vi "Sandbox.vi"() -> ()   [LabVIEW 2019, in "FPGA API Concrete.lvclass"]
uses:
  FPGA API Concrete.lvclass
  FPGA/TypeDef/DO index.ctl
  FPGA API Concrete.lvclass/FPGA API Concrete.ctl
  <vilib>/Utility/error.llb/Error Cluster From Error Code.vi
  <vilib>/rvi/errors/niLvFpgaAdjustHostInterfaceError.vi
  <vilib>/rvi/interface/nirviReadWriteControl/nirviReadWriteControl.xnode
  FPGA Ref.ctl
  <vilib>/ptbypt/NI_PtbyPt.lvlib
  NiFpgaLv.dll
  <vilib>/rvi/interface/Simulation/niFpgaSimulationCallBeginRW.vi
panel:
  in  "Mod5/AO1":fxp<+/-,20,5>
  out "Mod5/AO1 out":fxp<+/-,20,5>
  out "Ds":bool[](array[boolean])
  in  "#DO":T1 items=["DO 0 [KP1] [M12]", "DO 1 [ON KP2] [M21]", "DO 2 [ON KP3] [M24]", "DO 3 [WATER Y18.1 [DO3]]", "DO 4 [WATER Y18.2 [DO4]]", "DO 5 [KP6 Y29.1 33.7]", "DO 6 [KP7 Y29.2 33.8]", "DO 7 [KP8 Y29.3 33.9]", "DO 8 [KP9 Y29.4  33.12]", "DO 9 [KP10 Y29.5 33.1]", "DO 10 [KP11 Y29.6 33.2]", "DO 11 [KP12 Y29.7  33.13]", "DO 12 [KP13 Y29.8  33.11]", "DO 13 [KP14 Y29.9 33.10]", "DO 14 [KP15 Y29.10  33.6]", "DO 15 [KP16 Y29.11  33.5]", "DO 16 [KP17 Y29.12  33.4]", "DO 17 [KP18 Y29.13 33.3]", "DO 18 [AIR KP19]", "DO 19 [STEP DRIVE EN KP20]", "DO 20 [KP21 Y44.1 OPEN]", "DO 21 [ KP22 Y44.1 CLOSE]", "DO 22 [ KP23 Y44.2 OPEN]", "DO 23", "DO 24 [STEP DRIVE 1]", "DO 25 [STEP DRIVE 2]"]
  out "Numeric":i32
  out "avr %":dbl
  out "Raw %":dbl
  out "Waveform Chart":dbl[][](graph)
  out "DIs":bool[](array[boolean])
  out "dt(tiks) DI loop":u32
  out "dt(tiks) DO loop":u32
  out "dt(tiks) AI loop":u32
  out "error out":errorcluster
  in  "set":bool
  in  "Time uSec":u32
  in  "value":bool
  in  "stop":bool
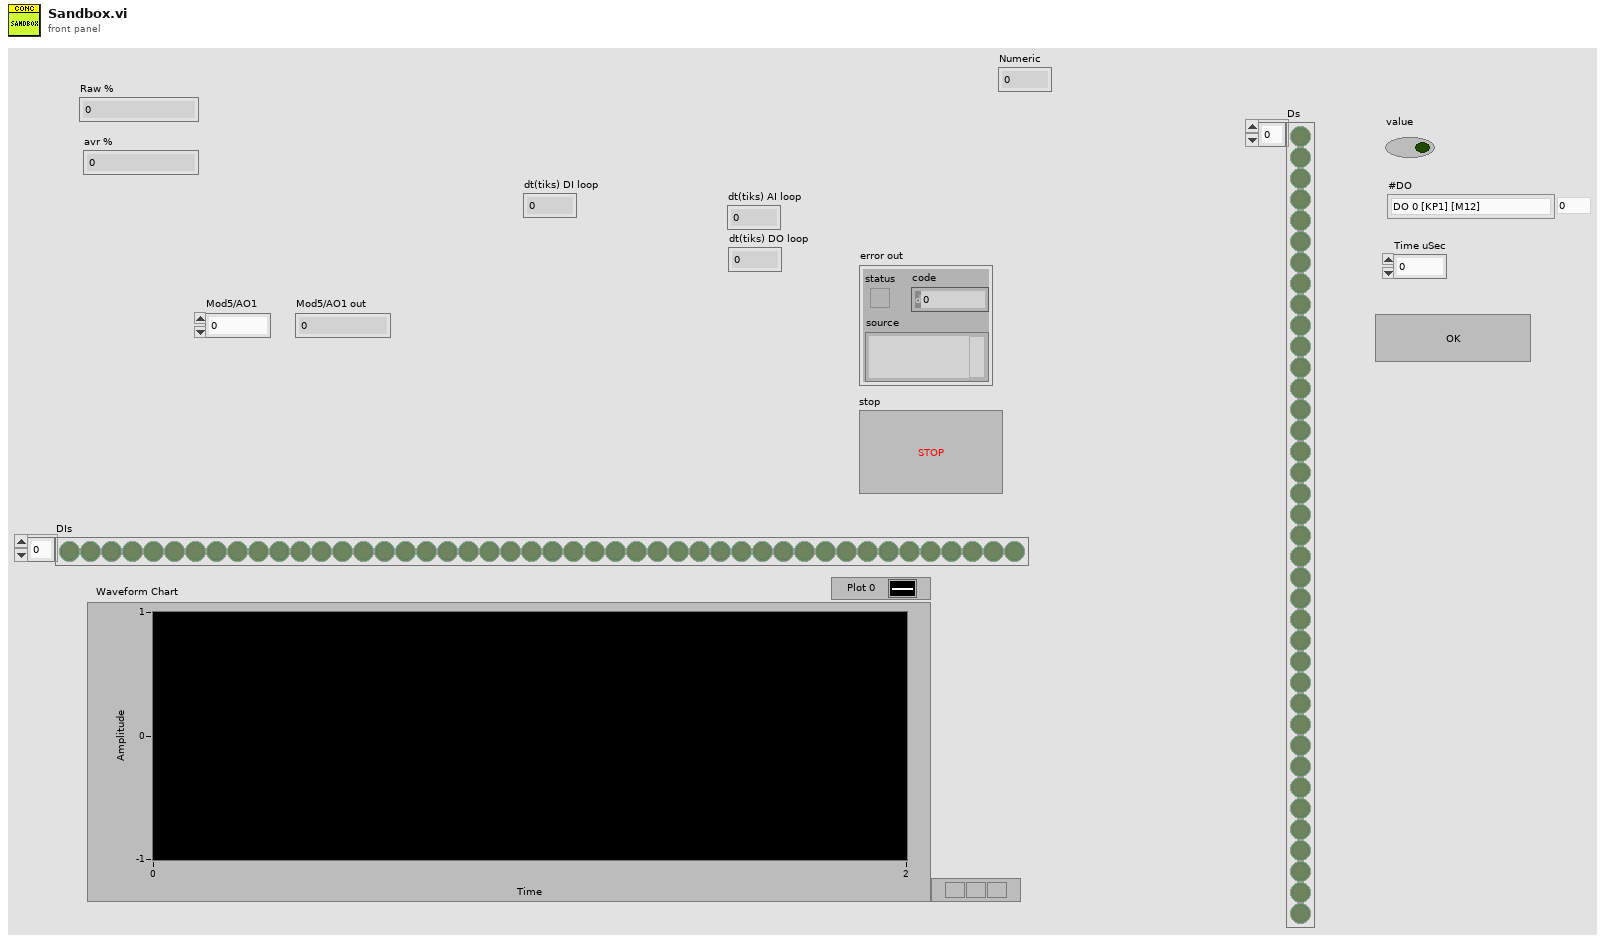
[diagram p1: front panel]
types:
  T1 = typedef "DO index.ctl" = u8
  T2 = typedef "FPGA API Concrete.lvclass/FPGA Ref.ctl" = refnum<k20>
  T3 = cluster{"AI_0 L5.1":fxp<+/-,21,-4>, "AI_1 T4.1":fxp<+/-,21,-4>, "AI_2 L5.2":fxp<+/-,21,-4>, "AI_3 T4.2":fxp<+/-,21,-4>, "AI_4 V":fxp<+/-,21,-4>, "AI_5 P38.1":fxp<+/-,21,-4>, "AI_6 P38.2":fxp<+/-,21,-4>, "AI_7 P38.3":fxp<+/-,21,-4>, "AI_8 P41.1":fxp<+/-,21,-4>, "AI_9 P41.2":fxp<+/-,21,-4>, "AI_10 P41.3":fxp<+/-,21,-4>, "AI_11":fxp<+/-,21,-4>, "AI_12":fxp<+/-,21,-4>, "AI_13":fxp<+/-,21,-4>, "AI_14":fxp<+/-,21,-4>, "AI_15":fxp<+/-,21,-4>}
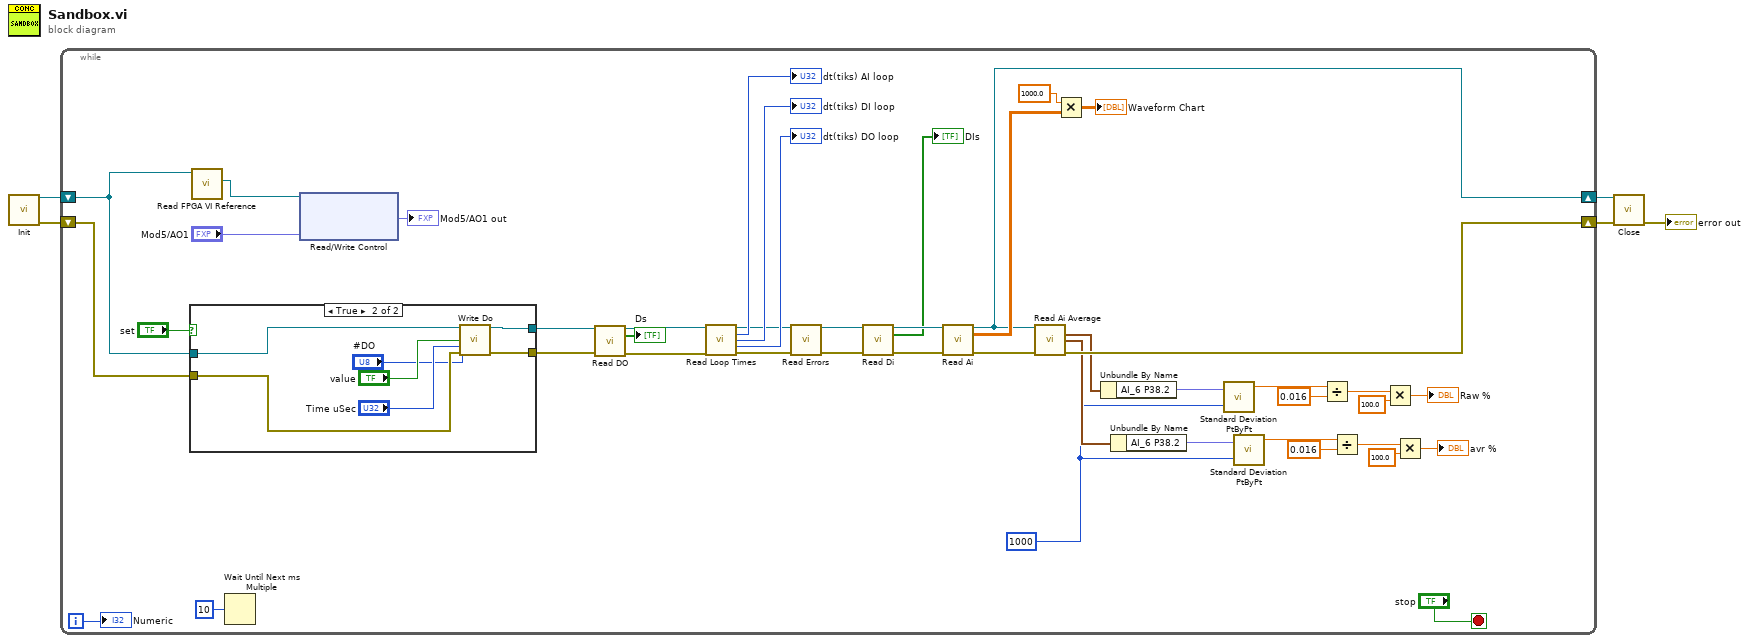
[diagram p0: block diagram]
diagram:
  n1 = call "Init.vi"() -> ("FPGA API out"=w5:refnum<class "FPGA API Concrete.lvclass">, "error out"=w4:errorcluster)  [unwired: 14 in]
  n2 = while {
    shift-right: [w34] -> w3
    shift-left: w5 -> [w9]
    shift-right: [w32] -> w2
    shift-left: w4 -> [w37]
    i -> [w16]
    stop <- "stop" stop-if-true
    w17 = 1000 ("sample length")
    n3 = case shown="True" "set" {
      tunnel: [w52 w59] -> w14
      tunnel: [w51 w58] -> w12
      tunnel: w9 -> [w52 w54]
      tunnel: w37 -> [w51 w57]
      frame False {
      }
      frame True {
        n4 = call-dynamic "Write Do.vi"("FPGA API in"=w54, "#DO"="#DO", "value"="value", "Time uSec"="Time uSec", "error in (no error)"=w57) -> ("FPGA API out"=w59:refnum<class "FPGA API Concrete.lvclass">, "error out"=w58:errorcluster)  [unwired: 9 in]
      }
    }
    n5 = call "Read FPGA VI Reference.vi"("FPGA API Concrete in"=w9) -> ("FPGA VI Reference"=w8:T2)  [unwired: 9 in, 1 out]
    n6 = Wait Until Next ms Multiple(millisecond multiple=u32 10) -> ()  [unwired: 1 out]
    n7 = xnode "Read/Write Control"("FPGA VI Reference In"=w8, "Mod5/AO1"="Mod5/AO1") -> ("Mod5/AO1 out"=→"Mod5/AO1 out":fxp<+/-,20,5>)  [unwired: 1 in, 2 out]
    n8 = call-dynamic "Read DO.vi"("FPGA API in"=w14, "error in (no error)"=w12) -> ("FPGA API out"=w13:refnum<class "FPGA API Concrete.lvclass">, "Ds"=→"Ds":bool[], "error out"=w11:errorcluster)  [unwired: 11 in]
    n9 = call-dynamic "Read Loop Times.vi"("FPGA API in"=w13, "error in (no error)"=w11) -> ("FPGA API out"=w43:refnum<class "FPGA API Concrete.lvclass">, "dt(tiks) AI loop"=→"dt(tiks) AI loop":u32, "dt(tiks) DI loop"=→"dt(tiks) DI loop":u32, "dt(tiks) DO loop"=→"dt(tiks) DO loop":u32, "error out"=w44:errorcluster)  [unwired: 8 in, 1 out]
    n10 = call-dynamic "Read Errors.vi"("FPGA API in"=w43, "error in (no error)"=w44) -> ("FPGA API out"=w42:refnum<class "FPGA API Concrete.lvclass">, "error out"=w41:errorcluster)  [unwired: 11 in, 1 out]
    n11 = call-dynamic "Read Di.vi"("FPGA API in"=w42, "error in (no error)"=w41) -> ("FPGA API out"=w39:refnum<class "FPGA API Concrete.lvclass">, "DIs"=→"DIs":bool[], "error out"=w40:errorcluster)  [unwired: 11 in]
    n12 = call-dynamic "Read Ai.vi"("FPGA API in"=w39, "error in (no error)"=w40) -> ("FPGA API out"=w34:refnum<class "FPGA API Concrete.lvclass">, "AI Data"=w36:dbl[][], "error out"=w33:errorcluster)  [unwired: 10 in, 1 out]
    n13 = call "Read Ai Average.vi"("FPGA API in"=w34, "error in (no error)"=w33) -> ("Raw"=w31:T3, "Average 1ms"=w18:T3, "error out"=w32:errorcluster)  [unwired: 10 in, 1 out]
    n14 = Multiply(x=1000.0, y=w36) -> (x*y=→"Waveform Chart":dbl[][])
    n15 = Unbundle By Name(w31) -> ("AI_6 P38.2"=w30:fxp<+/-,21,-4>)
    n16 = Unbundle By Name(w18) -> ("AI_6 P38.2"=w19:fxp<+/-,21,-4>)
    n17 = call <vilib>:"Standard Deviation PtByPt.vi"("x"=w30, "sample length"=w17) -> ("standard deviation"=w29:dbl)  [unwired: 1 in, 2 out]
    n18 = call <vilib>:"Standard Deviation PtByPt.vi"("x"=w19, "sample length"=w17) -> ("standard deviation"=w20:dbl)  [unwired: 1 in, 2 out]
    n19 = Divide(x=w29, y=0.016) -> (x/y=w27:dbl)
    n20 = Divide(x=w20, y=0.016) -> (x/y=w22:dbl)
    n21 = Multiply(x=w27, y=100.0) -> (x*y=→"Raw %":dbl)
    n22 = Multiply(x=w22, y=100.0) -> (x*y=→"avr %":dbl)
    "Numeric" <- w16
  }
  n23 = call-dynamic "Close.vi"("FPGA API in"=w3, "error in (no error)"=w2) -> ("error out"=→"error out":errorcluster)  [unwired: 12 in, 1 out]
